vi "Untitled 2 (SubVI).vi"(6 "Numeric 12":i32, 7 "Numeric 7":i32, 8 "Numeric 9":i32, 9 "Numeric 11":i32, 10 "Numeric 8":i32, 11 "Numeric 10":i32) -> (0 "Numeric 2":u8, 1 "Numeric 5":u8, 2 "Numeric 6":u8, 3 "Numeric":u8, 4 "Numeric 4":u8, 5 "Numeric 3":u8)   [LabVIEW 2014]
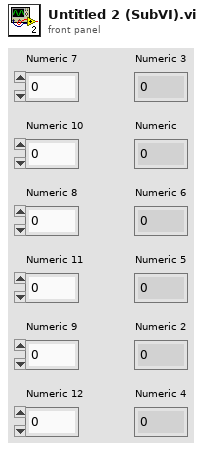
[diagram p1: front panel]
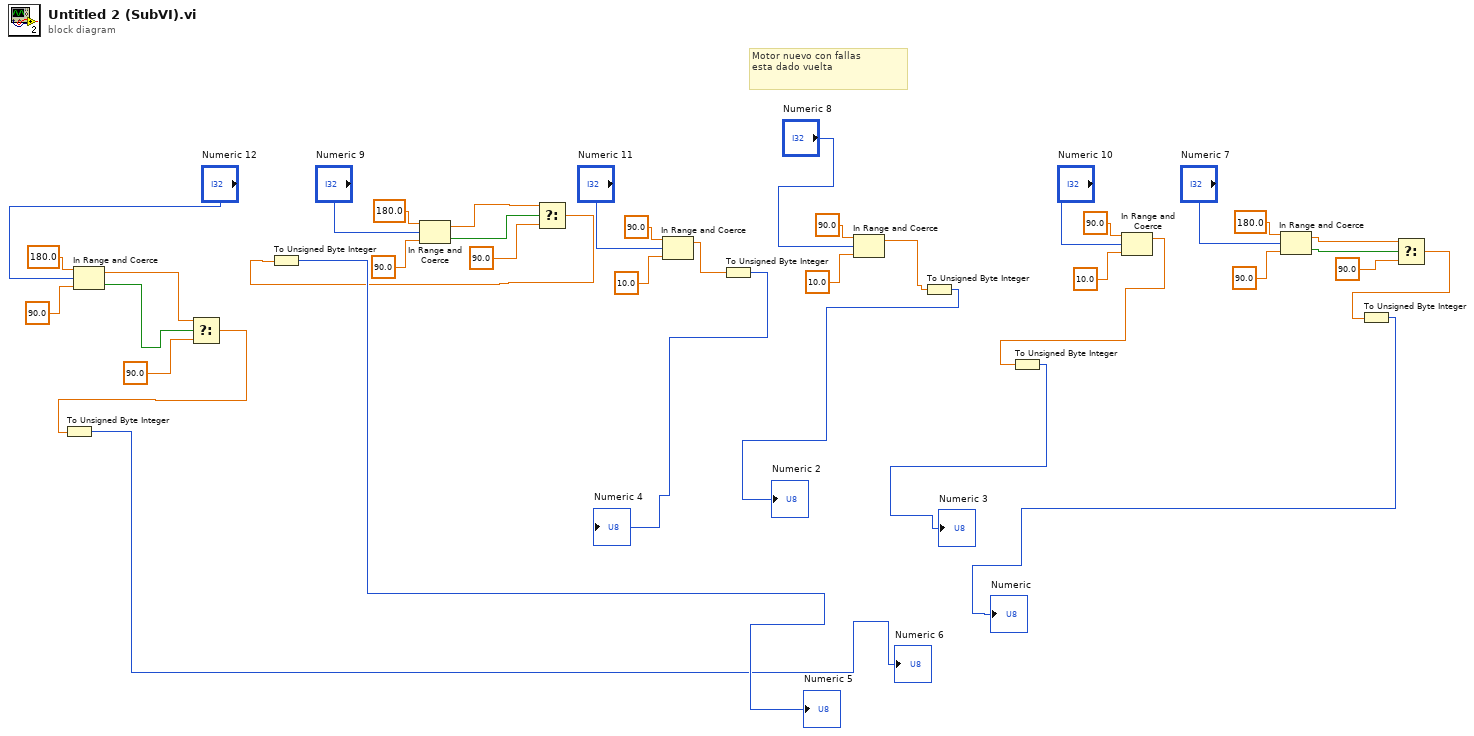
[diagram p0: block diagram]
diagram:
  # "Motor nuevo con fallas\nesta dado vuelta"
  n1 = In Range and Coerce(upper limit=180.0, x="Numeric 12", lower limit=90.0) -> (coerced(x)=w4:dbl, In Range?=w5:bool)
  n2 = Select(t=w4, s=w5, f=90.0) -> (s? t:f=w3:dbl)
  n3 = To Unsigned Byte Integer(number=w3) -> (unsigned 8bit integer=→"Numeric 6":u8)
  n4 = In Range and Coerce(upper limit=180.0, x="Numeric 9", lower limit=90.0) -> (coerced(x)=w32:dbl, In Range?=w31:bool)
  n5 = Select(t=w32, s=w31, f=90.0) -> (s? t:f=w30:dbl)
  n6 = To Unsigned Byte Integer(number=w30) -> (unsigned 8bit integer=→"Numeric 5":u8)
  n7 = In Range and Coerce(upper limit=90.0, x="Numeric 11", lower limit=10.0) -> (coerced(x)=w23:dbl)  [unwired: 1 out]
  n8 = To Unsigned Byte Integer(number=w23) -> (unsigned 8bit integer=→"Numeric 4":u8)
  n9 = In Range and Coerce(upper limit=90.0, x="Numeric 8", lower limit=10.0) -> (coerced(x)=w1:dbl)  [unwired: 1 out]
  n10 = To Unsigned Byte Integer(number=w1) -> (unsigned 8bit integer=→"Numeric 2":u8)
  n11 = In Range and Coerce(upper limit=90.0, x="Numeric 10", lower limit=10.0) -> (coerced(x)=w24:dbl)  [unwired: 1 out]
  n12 = To Unsigned Byte Integer(number=w24) -> (unsigned 8bit integer=→"Numeric 3":u8)
  n13 = In Range and Coerce(upper limit=180.0, x="Numeric 7", lower limit=90.0) -> (coerced(x)=w26:dbl, In Range?=w25:bool)
  n14 = Select(t=w26, s=w25, f=90.0) -> (s? t:f=w28:dbl)
  n15 = To Unsigned Byte Integer(number=w28) -> (unsigned 8bit integer=→"Numeric":u8)
